vi "Get Depth Image.vi"(6 "error in (no error)":errorcluster, 7 "Wait For Next Image?":bool=TRUE, 9 "in cluster":T1) -> (0 "error out":errorcluster, 2 "Depth Image":T2(plugin-control), 3 "out cluster":T1)   [LabVIEW 2011]
uses:
  <vilib>/vision/Image Controls.llb/IMAQ Image.ctl
  Microsoft.Kinect
panel:
  out "Image Is New?":bool
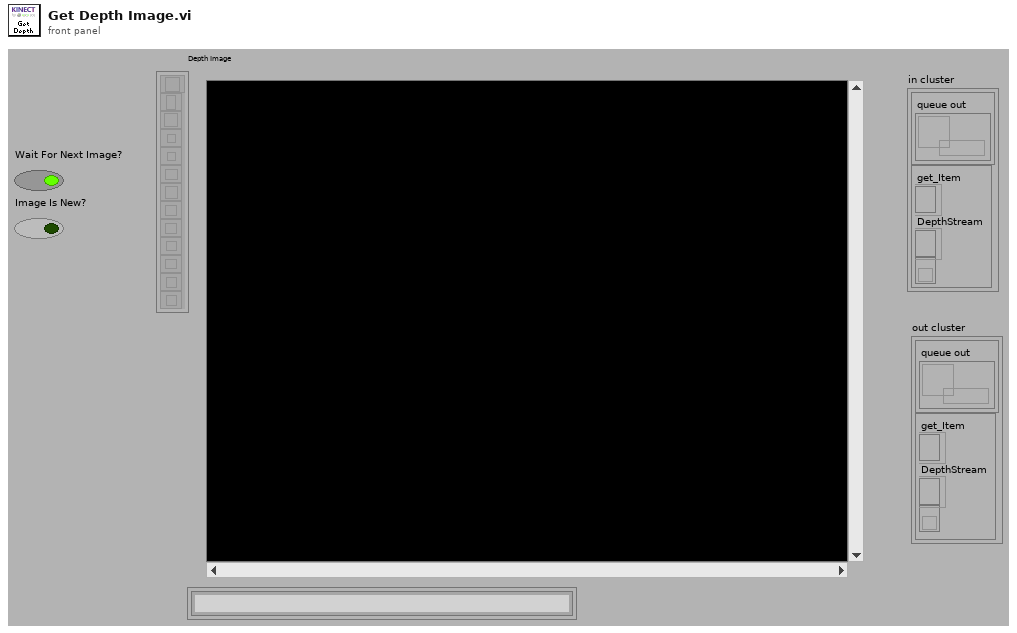
[diagram p1: front panel]
types:
  T1 = cluster{cluster{"queue out":refnum<queue>}, cluster{"get_Item":refnum<k24>, "DepthStream":refnum<k24>, "Event Callback":refnum<k27>}}
  T2 = typedef "IMAQ Image.ctl" = refnum<image>
  T3 = typedef "Image Type" = u32
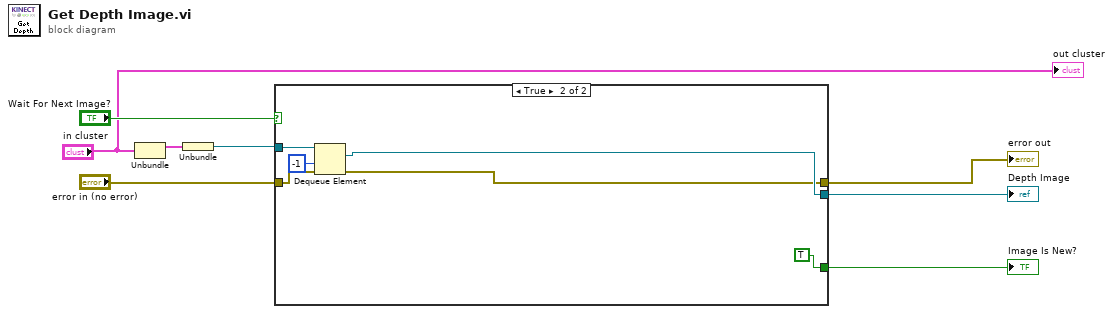
[diagram p0: block diagram]
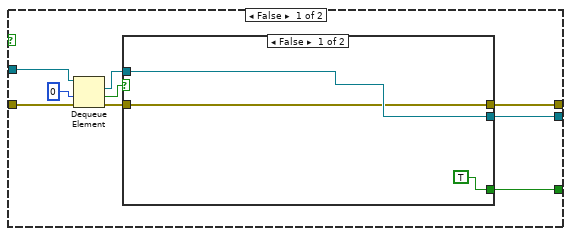
[diagram p2: hidden frame]
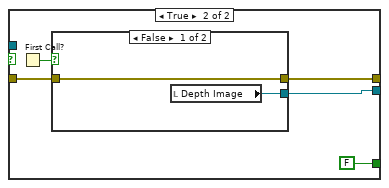
[diagram p3: hidden frame]
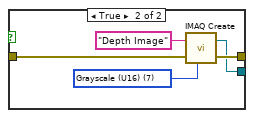
[diagram p4: hidden frame]
diagram:
  n1 = Unbundle("in cluster") -> (w4:cluster{"queue out":refnum<queue>})  [unwired: 1 out]
  n2 = Unbundle(w4) -> ("queue out"=w3:refnum<queue>)
  n3 = case shown="True" "Wait For Next Image?" {
    tunnel: "error in (no error)" -> [w13 w38]
    tunnel: [w15 w34] -> w5
    tunnel: [w16 w33] -> w1
    tunnel: [w17 TRUE] -> w8
    tunnel: w3 -> [w14 w36]
    frame False {
      n4 = Dequeue Element(queue=w14, timeout in ms (-1)=0, error in (no error)=w13) -> (element=w9:T2, timed out?=w10:bool, error out=w12:errorcluster)  [unwired: 1 out]
      n5 = case shown="False" w10 {
        tunnel: [w19 w23] -> w15
        tunnel: w12 -> [w18 w22]
        tunnel: [w18 w21] -> w16
        tunnel: [TRUE FALSE] -> w17
        tunnel: w9 -> [w19 _]
        frame False {
        }
        frame True {
          n6 = First Call?() -> (First Call?: T/F=w24:bool)
          n7 = case shown="False" w24 {
            tunnel: [w27 w28] -> w23
            tunnel: w22 -> [w26 w30]
            tunnel: [w26 w29] -> w21
            frame False {
              n8 = local read "Depth Image"() -> (w27:T2)
            }
            frame True {
              w31 = T3 7 items=["Grayscale (U8)", "Grayscale (I16)", "Grayscale (SGL)", "Complex (CSG)", "RGB (U32)", "HSL (U32)", "RGB (U64)", "Grayscale (U16)"] ("Image Type")
              n9 = call "IMAQ Create"("Image Name"="Depth Image", "Image Type"=w31, "error in (no error)"=w30) -> ("New Image"=w28:T2, "error out"=w29:errorcluster)  [unwired: 2 in]
            }
          }
        }
      }
    }
    frame True {
      n10 = Dequeue Element(queue=w36, timeout in ms (-1)=-1, error in (no error)=w38) -> (element=w34:T2, error out=w33:errorcluster)  [unwired: 2 out]
    }
  }
  "Depth Image" <- w5
  "error out" <- w1
  "Image Is New?" <- w8
  "out cluster" <- "in cluster"
